vi "VzScanSettingsHandler.vi"(9 "Vz Counter":i16, 10 "Digitizer Settings in":T1 {"Trigger Settings"."Trig Slope" items=["Positive", "Negative"]; "Trigger Settings"."Level (mV)" format="%.2f"; "Trigger Settings"."Trig Coupling" items=["DC 1 MOhm", "AC 1 MOhm", "DC 50 Ohm", "AC 50 Ohm"]; "Trigger Settings"."Trig Source" items=["Chan 1", "External"]; "Rel Dig Delay" format="%.2f"; "DigTimeOut" format="%.2f"; "Avg Num" min=1; "Offset delay (us)" format="%.2f"; "Additional dig delay (us)" format="%.2f"; "Digitizer delay (us)" format="%.2f"}, 11 "Length of all Planes (mm)":refnum<vi>) -> (1 "Digitizer Settings out":T1 {"Trigger Settings"."Trig Slope" items=["Positive", "Negative"]; "Trigger Settings"."Level (mV)" format="%.2f"; "Trigger Settings"."Trig Coupling" items=["DC 1 MOhm", "AC 1 MOhm", "DC 50 Ohm", "AC 50 Ohm"]; "Trigger Settings"."Trig Source" items=["Chan 1", "External"]; "Rel Dig Delay" format="%.2f"; "DigTimeOut" format="%.2f"; "Avg Num" min=1; "Offset delay (us)" format="%.2f"; "Additional dig delay (us)" format="%.2f"; "Digitizer delay (us)" format="%.2f"}, 2 "rf points per line Temp":i32, 3 "Additional dig delay (us) Temp":dbl, 4 "Length of\nall planes (mm) Temp":dbl=128.0 format="%.2f", 5 "Digitizer delay (us) (Temp)":dbl, 6 "LC read pt offset temp":dbl)   [LabVIEW 2022 SP3]
uses:
  Digitizers/-DigitizerRoutines/DigitizerSettings.ctl
  Digitizers/-DigitizerRoutines/Digitizer.ctl
  Digitizers/-DigitizerRoutines/DigConfig.ctl
  Digitizers/-DigitizerRoutines/DigitizerID.ctl
  C:/Windows/System32/ADQAPI_dotNet_helper.dll
  Motion Controllers/-MotionRoutines/MotionGlobals.vi
  <instrlib>/LeCroy Wave Series/LeCroy Wave Series.lvlib
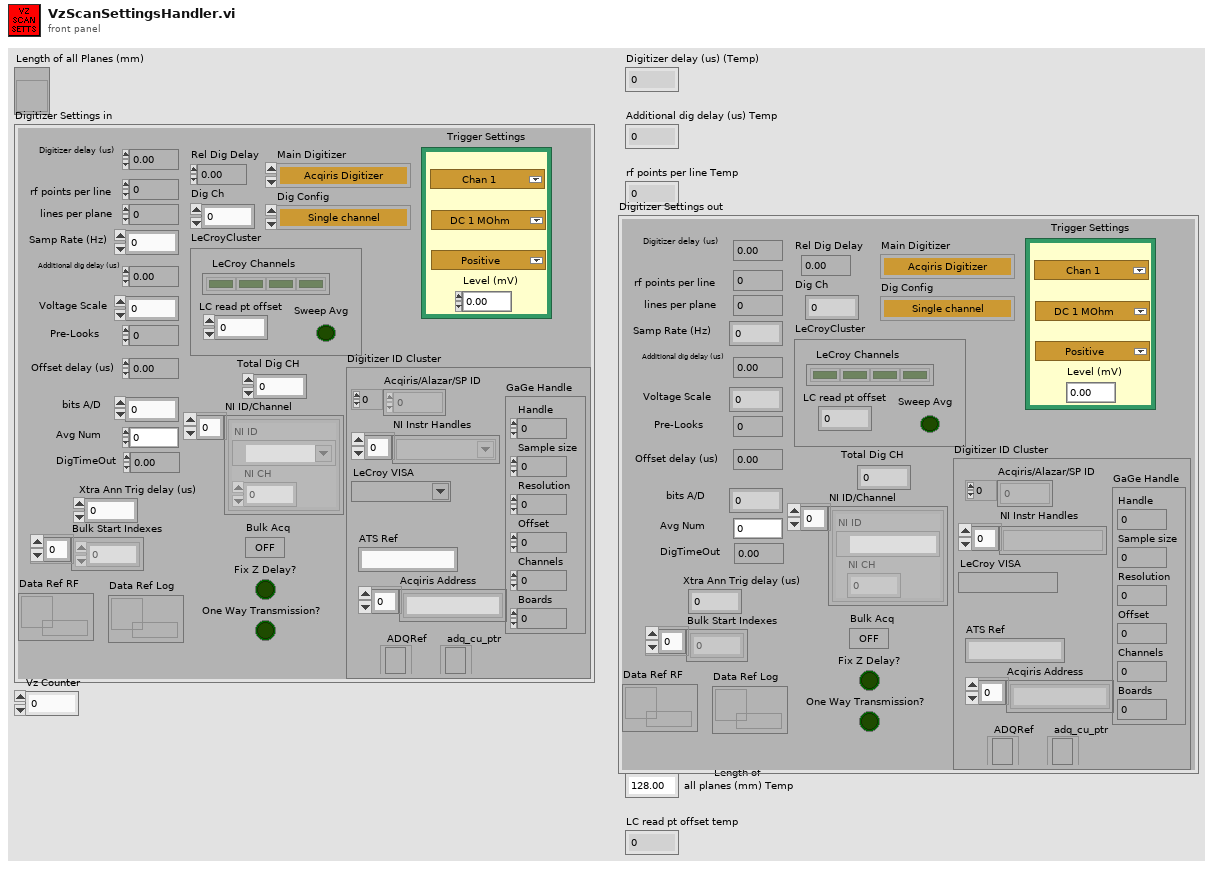
[diagram p1: front panel]
types:
  T1 = typedef "DigitizerSettings.ctl" = cluster{"Digitizer delay (us) ":dbl, "rf points per line":i32, "lines per plane":i32, "Samp Rate (Hz)":dbl, "Additional dig delay (us)":dbl, "Voltage Scale":dbl, "Pre-Looks":i32, "Offset delay (us)":dbl, "bits A/D":i8, "Avg Num":i32, "DigTimeOut":sgl, "Rel Dig Delay":sgl, "Dig Ch":i32, "LeCroyCluster":cluster{"LeCroy Channels":bool[], "LC read pt offset":dbl, "Sweep Avg":bool}, "Main Digitizer":T2, "Dig Config":T3, "Digitizer ID Cluster":T4, "Trigger Settings":cluster{"Trig Source":u16, "Trig Coupling":u16, "Trig Slope":u16, "Level (mV)":dbl}, "Bulk Acq":bool, "Bulk Start Indexes":i32[], "Data Ref RF":refnum<data-value>, "NI ID/Channel":cluster{"NI ID":refnum<k15>, "NI CH":i32}[], "Total Dig CH":i32, "Xtra Ann Trig delay (us)":dbl, "Fix Z Delay?":bool, "One Way Transmission?":bool, "Data Ref Log":refnum<data-value>}
  T2 = typedef "Digitizer.ctl" = enum16{"Acqiris Digitizer", "NI Digitizer", "LeCroy", "GaGe", "AlazarTech", "No Digitizer", "Teledyne"}
  T3 = typedef "DigConfig.ctl" = enum16{"Single channel", "2 Chans w/ 2 Acqiris", "2 Chans w/ 1 Acqiris", "5-CH Pulser New", "5-CH pulser w/ ann array", "5-pass style ann array", "Empty"}
  T4 = typedef "DigitizerID.ctl" = cluster{"Acqiris/Alazar/SP ID":u32[], "NI Instr Handles":refnum<k15>[], "LeCroy VISA":refnum<visa-resource-name>, "GaGe Handle":cluster{"Handle":u32, "Sample size":u32, "Resolution":i32, "Offset":i32, "Channels":u32, "Boards":u32}, "ATS Ref":string, "Acqiris Address":string[], "ADQRef":refnum<k24>, "adq_cu_ptr":refnum<k24>}
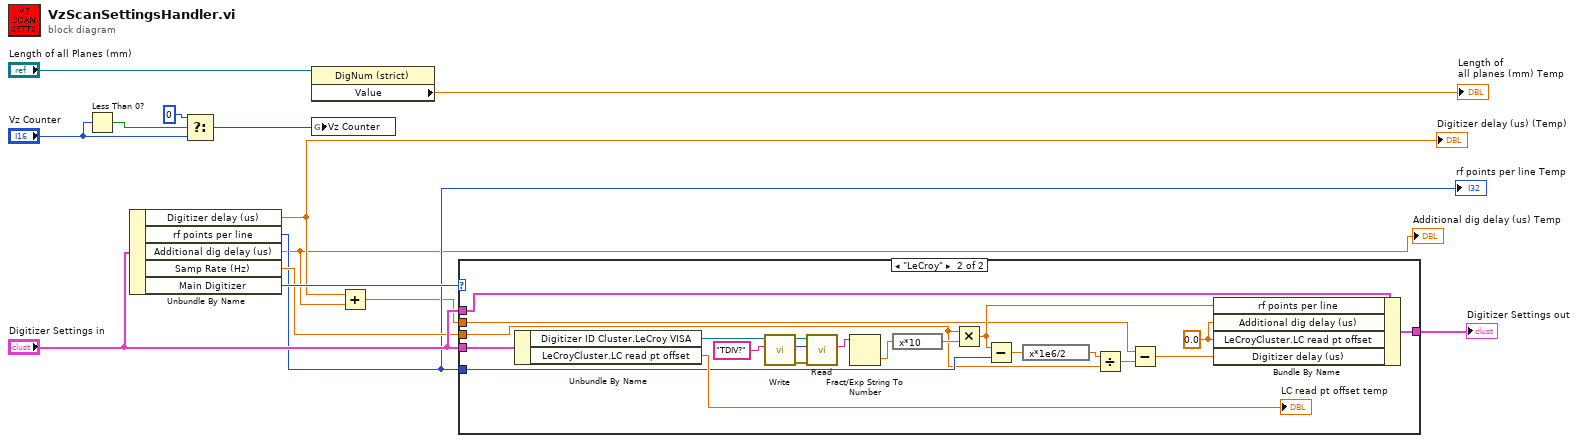
[diagram p0: block diagram]
diagram:
  n1 = Less Than 0?(x="Vz Counter") -> (x < 0?=w3:bool)
  n2 = Unbundle By Name("Digitizer Settings in") -> ("Digitizer delay (us)"=w6:dbl, "rf points per line"=w8:i32, "Additional dig delay (us)"=w5:dbl, "Samp Rate (Hz)"=w9:dbl, "Main Digitizer"=w10:T2)
  "Additional dig delay (us) Temp" <- w5
  "rf points per line Temp" <- w8
  "Digitizer delay (us) (Temp)" <- w6
  n3 = Select(t=i16 0, s=w3, f="Vz Counter") -> (s? t:f=w1:i16)
  n4 = property on="Property Node" class="DigNum (strict)"(reference="Length of all Planes (mm)") -> ("Value"=→"Length of\nall planes (mm) Temp":dbl)  [unwired: 1 in, 2 out]
  n5 = global write "MotionGlobals.vi" "Vz Counter"(w1) -> ()
  n6 = Add(x=w6, y=w5) -> (x+y=w4:dbl)
  n7 = case shown="\"LeCroy\"" w10 {
    tunnel: "Digitizer Settings in" -> [_ w32]
    tunnel: w9 -> [_ w20]
    tunnel: "Digitizer Settings in" -> [w15 w27]
    tunnel: [w15 w26] -> w14
    tunnel: w8 -> [_ w22]
    tunnel: w4 -> [_ w16]
    frame "Acqiris Digitizer", Default {
    }
    frame "LeCroy" {
      w24 = 0.0 ("Additional dig delay (us)")
      n8 = Unbundle By Name(w32) -> ("Digitizer ID Cluster.LeCroy VISA"=w31:refnum<visa-resource-name>, "LeCroyCluster.LC read pt offset"=→"LC read pt offset temp":dbl)
      n9 = call <instrlib>:"Write.vi"("Write Buffer"="TDIV?", "VISA resource name"=w31) -> ("error out"=w36:errorcluster, "Return Count"=w30:u32, "VISA resource name out"=w35:refnum<visa-resource-name>)  [unwired: 7 in]
      n10 = call <instrlib>:"Read.vi"("error in (no error)"=w36, "Byte Count"=w30, "VISA resource name"=w35) -> ("Read Buffer"=w33:string)  [unwired: 5 in, 3 out]
      n11 = Fract/Exp String To Number(string=w33) -> (number=w29:dbl)  [unwired: 3 in, 1 out]
      n12 = expression code="x*10"(w29) -> (w28:dbl)
      n13 = Multiply(x=w20, y=w28) -> (x*y=w23:dbl)
      n14 = Subtract(x=w23, y=w22) -> (x-y=w21:dbl)
      n15 = expression code="x*1e6/2"(w21) -> (w19:dbl)
      n16 = Divide(x=w19, y=w20) -> (x/y=w17:dbl)
      n17 = Subtract(x=w16, y=w17) -> (x-y=w18:dbl)
      n18 = Bundle By Name(cluster=w27, "rf points per line"=w23, "Additional dig delay (us)"=w24, "LeCroyCluster.LC read pt offset"=w24, "Digitizer delay (us)"=w18) -> (w26:T1)
    }
  }
  "Digitizer Settings out" <- w14
